vi "Choreo_TrajectoryDifferential_GetInitialSample.vi"(9 "mirrorForRedAlliance":bool, 11 "ChoreoTrajectoryDifferential":T2) -> (1 "Exists":bool, 3 "sample":T1={"timestamp"=-999.0, "x"=0.0, "y"=0.0, "heading"=0.0, "velocityL"=0.0, "velocityR"=0.0, "angularVelocity"=0.0, "accelL"=0.0, "accelR"=0.0, "accelAngular"=0.0, "forceL"=0.0, "forceR"=0.0})   [LabVIEW 2019, in "ChoreoLib.lvlib"]
doc: "Returns the first swerve sample in the trajectory.\n \nThis function will return empty and Exists will be false.\n \nInputs: \n -- ChoreoTrajectorySwerve - cluster - data cluster for this trajectory \n -- mirrorForRedAlliance - boolean - whether or not to return the sample as mirrored across the field\n\nOutputs: \n -- Sample - cluster - The first swerve sample in the trajectory.\n -- exists - boolean - the sample exits."
uses:
  ChoreoLib.lvlib
  TypeDef/ChoreoTrajectoryDifferential.ctl
  TypeDef/ChoreoDifferentialSample.ctl
  TypeDef/ChoreoEventMarker.ctl
  Choreo_Util_AllianceFlipGetFlipper.vi
  Choreo_Util_AllianceFlipX.vi
  Choreo_Util_AllianceFlipY.vi
  Choreo_Util_AllianceFlipHeading.vi
  Choreo_DifferentialSample_New.vi
  Choreo_Choreo_Globals.vi
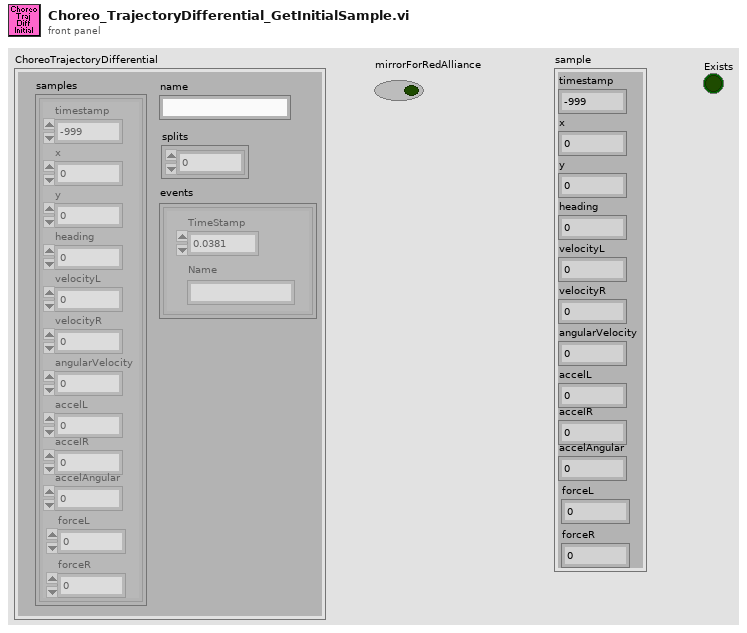
[diagram p1: front panel]
types:
  T1 = typedef "ChoreoLib.lvlib/ChoreoDifferentialSample.ctl" = cluster{"timestamp":dbl, "x":dbl, "y":dbl, "heading":dbl, "velocityL":dbl, "velocityR":dbl, "angularVelocity":dbl, "accelL":dbl, "accelR":dbl, "accelAngular":dbl, "forceL":dbl, "forceR":dbl}
  T2 = typedef "ChoreoLib.lvlib/ChoreoTrajectoryDifferential.ctl" = cluster{"name":string, "samples":T1[], "splits":i32[], "events":T3[]}
  T3 = typedef "ChoreoLib.lvlib/ChoreoEventMarker.ctl" = cluster{"TimeStamp":dbl, "Name":string}
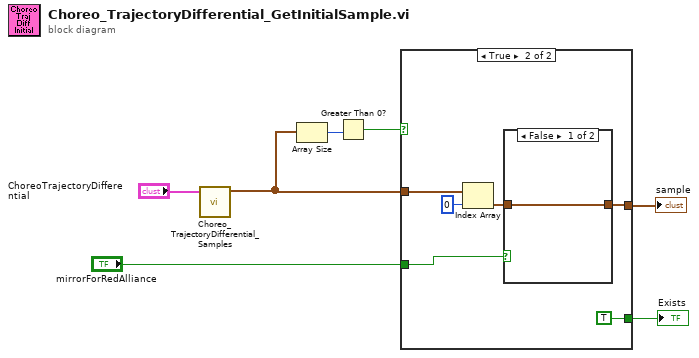
[diagram p0: block diagram]
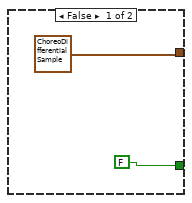
[diagram p2: hidden frame]
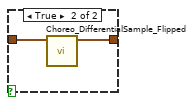
[diagram p3: hidden frame]
diagram:
  n1 = call "Choreo_TrajectoryDifferential_Samples.vi"("ChoreoTrajectoryDifferential"="ChoreoTrajectoryDifferential") -> ("samples"=w4:T1[])  [unwired: 10 in]
  n2 = Array Size(array=w4) -> (size(s)=w7:i32)
  n3 = Greater Than 0?(x=w7) -> (x > 0?=w6:bool)
  n4 = case shown="True" w6 {
    tunnel: w4 -> [_ w15]
    tunnel: [T1 {"timestamp"=-999.0, "x"=0.0, "y"=0.0, "heading"=0.0, "velocityL"=0.0, "velocityR"=0.0, "angularVelocity"=0.0, "accelL"=0.0, "accelR"=0.0, "accelAngular"=0.0, "forceL"=0.0, "forceR"=0.0} ("samples") w10] -> w2
    tunnel: [FALSE TRUE] -> w3
    tunnel: "mirrorForRedAlliance" -> [_ w12]
    frame False {
    }
    frame True {
      n5 = Index Array(array=w15, index=0) -> (element=w11:T1)
      n6 = case shown="False" w12 {
        tunnel: [w16 w17] -> w10
        tunnel: w11 -> [w16 w18]
        frame False {
        }
        frame True {
          n7 = call "Choreo_DifferentialSample_Flipped.vi"("ChoreoDifferentialSample"=w18) -> ("FlippedDifferentialSample"=w17:T1)  [unwired: 10 in]
        }
      }
    }
  }
  "Exists" <- w3
  "sample" <- w2
